vi "Code Cleanup.vi"() -> ()   [LabVIEW 2023]
panel:
  out "Array":path[](array[path])
  in  "stop":bool
  out "Current VI":string
  out "Status":string
  in  "Action":T1(ring)
  in  "root path":path
  out "error out":errorcluster
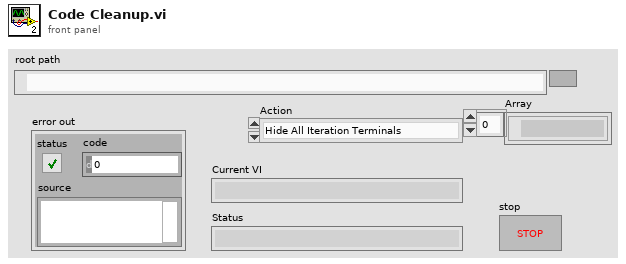
[diagram p1: front panel]
types:
  T1 = enum16{"Hide All Iteration Terminals", "Rename Window Title to VI Name", "Set Minimum Pane Size to (0,0)", "Set Origin to (0,0)", "Set Terminals to Required", "Fix VI Icon Properties", "Remove Autogrow from Structures", "Arrange Control Labels", "Format Control Labels", "Set Default FP BG Color", "Unshow Controls as Icons", "Set Modern Control Style"}
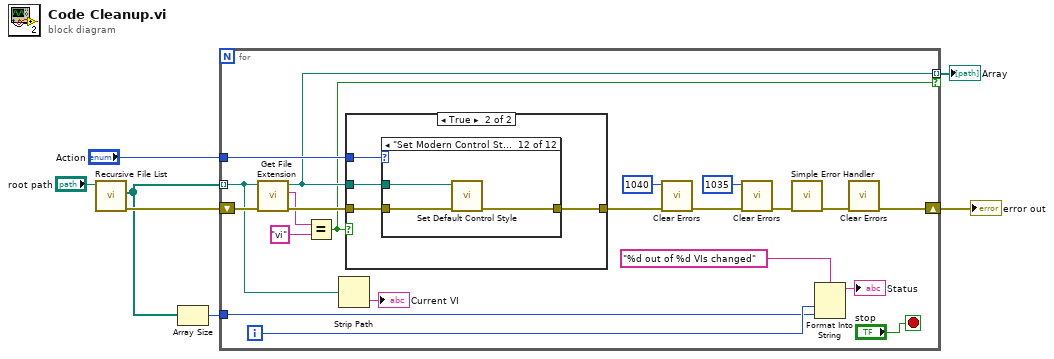
[diagram p0: block diagram]
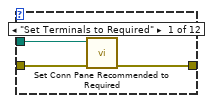
[diagram p3: hidden frame]
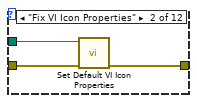
[diagram p4: hidden frame]
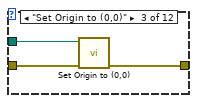
[diagram p5: hidden frame]
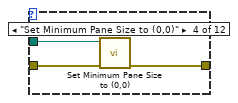
[diagram p6: hidden frame]
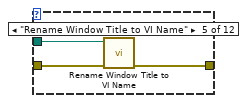
[diagram p7: hidden frame]
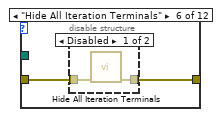
[diagram p8: hidden frame]
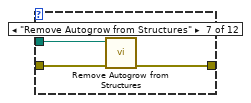
[diagram p10: hidden frame]
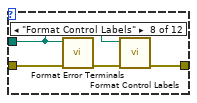
[diagram p11: hidden frame]
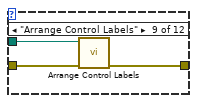
[diagram p12: hidden frame]
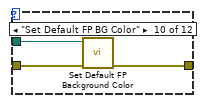
[diagram p13: hidden frame]
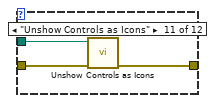
[diagram p14: hidden frame]
diagram:
  n1 = call <vilib>:"Recursive File List.vi"("Folder Path"="root path") -> ("error out"=w7:errorcluster, "All Files in Dir"=w3:path[])  [unwired: 6 in, 3 out]
  n2 = Array Size(array=w3) -> (size(s)=w2:i32)
  n3 = for {
    tunnel: w3 -> [w11] mode=indexing
    shift-right: [w21] -> w6
    shift-left: w7 -> [w28]
    tunnel: "Action" -> [w24]
    tunnel: w2 -> [w9]
    tunnel: [w19] -> w1 mode=indexing if=w18
    i -> [w10]
    stop <- "stop" stop-if-true
    n4 = call <vilib>:"Get File Extension.vi"("error in (no error)"=w28, "file"=w11) -> ("error out"=w27:errorcluster, "lowercase file extension"=w26:string, "dup file"=w19:path)  [unwired: 5 in, 2 out]
    n5 = Equal?(x=w26, y="vi") -> (x = y?=w18:bool)
    n6 = Strip Path(path=w11) -> (name=→"Current VI":string)  [unwired: 1 out]
    n7 = case shown="True" w18 {
      tunnel: w27 -> [w29 w33]
      tunnel: w19 -> [_ w32]
      tunnel: [w29 w31] -> w22
      tunnel: w24 -> [_ w30]
      frame False {
      }
      frame True {
        n8 = case shown="\"Set Modern Control Style\"" w30 {
          tunnel: w33 -> [w36 w39 w42 w45 w48 w50 w56 w59 w63 w66 w69 w72]
          tunnel: w32 -> [w35 w37 w40 w43 w46 _ w54 w57 w61 w64 w67 w70]
          tunnel: [w34 w38 w41 w44 w47 w49 w55 w60 w62 w65 w68 w71] -> w31
          frame "Set Terminals to Required" {
            n9 = call "Set Conn Pane Recommended to Required.vi"("error in (no error)"=w36, "vi path"=w35) -> ("error out"=w34:errorcluster)  [unwired: 9 in]
          }
          frame "Fix VI Icon Properties" {
            n10 = call "Set Default VI Icon Properties.vi"("error in (no error)"=w39, "vi path"=w37) -> ("error out"=w38:errorcluster)  [unwired: 9 in]
          }
          frame "Set Origin to (0,0)" {
            n11 = call "Set Origin to (0,0).vi"("error in (no error)"=w42, "vi path"=w40) -> ("error out"=w41:errorcluster)  [unwired: 9 in]
          }
          frame "Set Minimum Pane Size to (0,0)" {
            n12 = call "Set Minimum Pane Size to (0,0).vi"("error in (no error)"=w45, "vi path"=w43) -> ("error out"=w44:errorcluster)  [unwired: 9 in]
          }
          frame "Rename Window Title to VI Name" {
            n13 = call "Rename Window Title to VI Name.vi"("error in (no error)"=w48, "vi path"=w46) -> ("error out"=w47:errorcluster)  [unwired: 9 in]
          }
          frame "Hide All Iteration Terminals" {
            n14 = disable-structure shown="Disabled" {
              disable-tunnel: w50 -> [w52 w53]
              disable-tunnel: [w51 w53] -> w49
              frame Disabled {
                n15 = call "Hide All Iteration Terminals.vi"("error in (no error)"=w52) -> ("error out"=w51:errorcluster)  [unwired: 9 in, 1 out]
              }
              frame Enabled {
              }
            }
          }
          frame "Remove Autogrow from Structures" {
            n16 = call "Remove Autogrow from Structures.vi"("error in (no error)"=w56, "vi path"=w54) -> ("error out"=w55:errorcluster)  [unwired: 9 in]
          }
          frame "Format Control Labels" {
            n17 = call "Format Error Terminals.vi"("error in (no error)"=w59, "vi path"=w57) -> ("error out"=w58:errorcluster)  [unwired: 9 in]
            n18 = call "Format Control Labels.vi"("error in (no error)"=w58, "vi path"=w57) -> ("error out"=w60:errorcluster)  [unwired: 9 in]
          }
          frame "Arrange Control Labels" {
            n19 = call "Arrange Control Labels.vi"("error in (no error)"=w63, "vi path"=w61) -> ("error out"=w62:errorcluster)  [unwired: 9 in]
          }
          frame "Set Default FP BG Color" {
            n20 = call "Set Default FP Background Color.vi"("error in (no error)"=w66, "vi path"=w64) -> ("error out"=w65:errorcluster)  [unwired: 9 in]
          }
          frame "Unshow Controls as Icons" {
            n21 = call "Unshow Controls as Icons.vi"("error in"=w69, "vi path"=w67) -> ("error out"=w68:errorcluster)  [unwired: 9 in]
          }
          frame "Set Modern Control Style" {
            n22 = call "Set Default Control Style.vi"("error in (no error)"=w72, "vi path"=w70) -> ("error out"=w71:errorcluster)  [unwired: 9 in]
          }
        }
      }
    }
    n23 = call <vilib>:"Clear Errors.vi"("error in (no error)"=w22, "specific error code to clear (0: all)"=1040) -> ("error out"=w16:errorcluster)  [unwired: 4 in, 1 out]
    n24 = call <vilib>:"Clear Errors.vi"("error in (no error)"=w16, "specific error code to clear (0: all)"=1035) -> ("error out"=w15:errorcluster)  [unwired: 4 in, 1 out]
    n25 = call <vilib>:"Simple Error Handler.vi"("error in (no error)"=w15) -> ("error out"=w23:errorcluster)  [unwired: 4 in, 4 out]
    n26 = Format Into String(format string="%d out of %d VIs changed", w10, w9) -> (resulting string=→"Status":string)  [unwired: 2 in, 1 out]
    n27 = call <vilib>:"Clear Errors.vi"("error in (no error)"=w23) -> ("error out"=w21:errorcluster)  [unwired: 5 in, 1 out]
  }
  "error out" <- w6
  "Array" <- w1
